vi "ics_ids_save_2D.vi"(0 "pixels":i32, 1 "filename":string, 3 "folder":path=path "D:/User/Sergey/ids_ics_trainer", 5 "Dwell":dbl, 7 "data":i32[][](array[numeric]), 9 "Range":dbl, 11 "error in":errorcluster) -> (4 "saved":bool, 15 "error out":errorcluster)   [LabVIEW 2009]
panel:
  out "text":string
  in  "scale I":i32=1
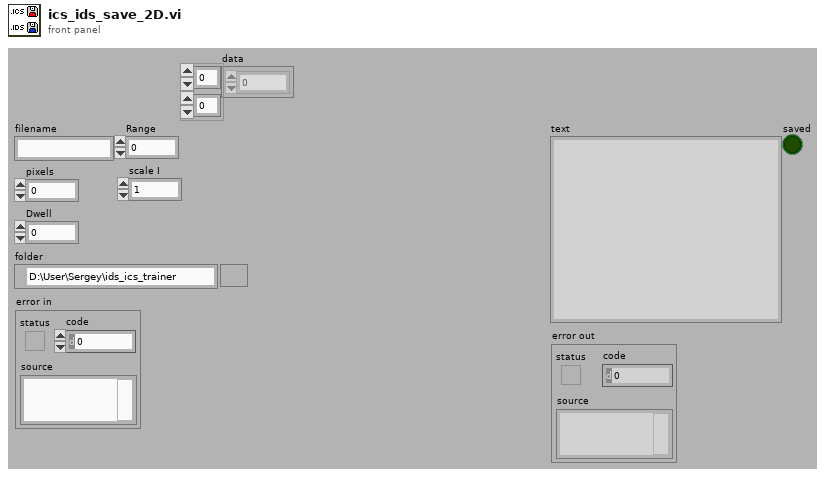
[diagram p1: front panel]
types:
  T1 = enum16{"open", "replace", "create", "open or create", "replace or create", "replace or create with confirmation"}
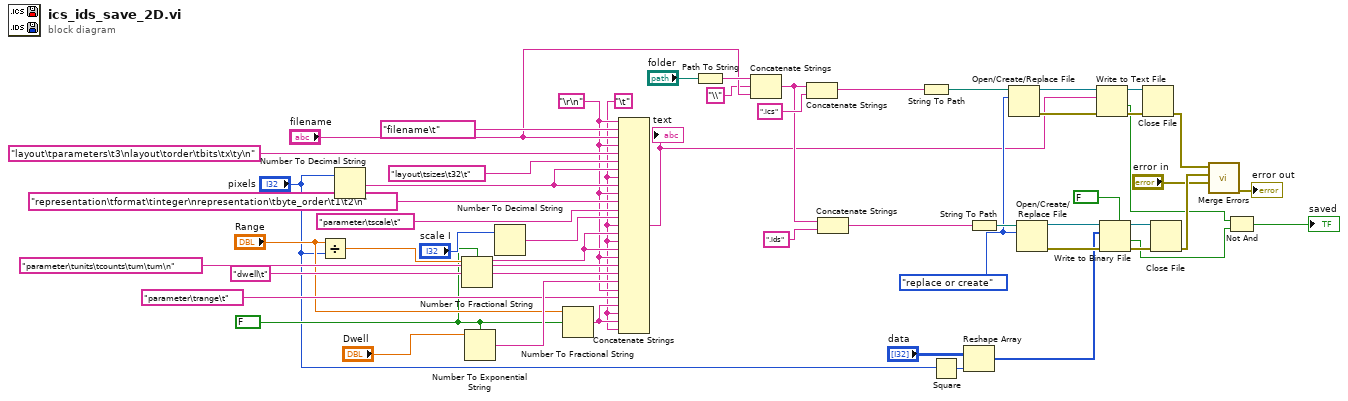
[diagram p0: block diagram]
diagram:
  w10 = FALSE ("use system decimal point (T)")
  w29 = T1."replace or create" ("operation (0:open)")
  w11 = "\t"
  w31 = "\r\n"
  n1 = Divide(x="Range", y="pixels") -> (x/y=w46:dbl)
  n2 = Number To Decimal String(number="pixels") -> (decimal integer string=w51:string)  [unwired: 1 in]
  n3 = Number To Fractional String(use system decimal point (T)=w10, number=w46) -> (F-format string=w45:string)  [unwired: 2 in]
  n4 = Number To Exponential String(number="Dwell", 1:w10) -> (E-format string=w40:string)  [unwired: 2 in]
  n5 = Number To Decimal String(number="scale I") -> (decimal integer string=w47:string)  [unwired: 1 in]
  n6 = Number To Fractional String(use system decimal point (T)=w10, number="Range") -> (F-format string=w12:string)  [unwired: 2 in]
  n7 = Concatenate Strings(w31, "filename\t" ("string"), "filename", w31, "layout\tparameters\t3\nlayout\torder\tbits\tx\ty\n" ("string"), "layout\tsizes\t32\t" ("string"), w51, w11, w51, w31, "representation\tformat\tinteger\nrepresentation\tbyte_order\t1\t2\n" ("string"), "parameter\tscale\t" ("string"), w47, w11, w45, w11, w45, w31, "parameter\tunits\tcounts\tum\tum\n" ("string"), "dwell\t" ("string"), w40, w31, "parameter\trange\t" ("string"), w12, w11, w12, w11) -> (w22:string)
  "text" <- w22
  n8 = Path To String(path="folder") -> (string=w35:string)
  n9 = Concatenate Strings(w35, "\\" ("string"), "filename") -> (w24:string)
  n10 = Concatenate Strings(w24, ".ics" ("string")) -> (w26:string)
  n11 = Concatenate Strings(w24, ".ids" ("string")) -> (w23:string)
  n12 = String To Path(string=w26) -> (path=w33:path)
  n13 = Square(x="pixels") -> (x^2=w16:i32)
  n14 = Reshape Array("data", w16) -> (w15:i32[])
  n15 = String To Path(string=w23) -> (path=w30:path)
  n16 = Open/Create/Replace File(file path (use dialog)=w33, operation (0:open)=w29) -> (refnum out=w37:refnum<file>, error out=w36:errorcluster)  [unwired: 4 in, 1 out]
  n17 = Open/Create/Replace File(file path (use dialog)=w30, operation (0:open)=w29) -> (refnum out=w19:refnum<file>, error out=w18:errorcluster)  [unwired: 4 in, 1 out]
  n18 = Write to Text File(file (use dialog)=w37, text=w22, error in=w36) -> (refnum out=w39:refnum<file>, cancelled=w5:bool, error out=w38:errorcluster)  [unwired: 1 in]
  n19 = Write to Binary File(file (use dialog)=w19, data=w15, error in=w18, 5:FALSE ("prepend array or string size? (T)")) -> (refnum out=w20:refnum<file>, cancelled=w4:bool, error out=w21:errorcluster)  [unwired: 2 in]
  n20 = Close File(refnum=w39, error in=w38) -> (error out=w9:errorcluster)  [unwired: 1 out]
  n21 = Close File(refnum=w20, error in=w21) -> (error out=w8:errorcluster)  [unwired: 1 out]
  n22 = call <vilib>:"Merge Errors.vi"("error in 3 (no error)"="error in", "error in 2 (no error)"=w8, "error in 1 (no error)"=w9) -> ("error out"=→"error out":errorcluster)  [unwired: 4 in]
  n23 = Not And(1:w4, 2:w5) -> (0:→"saved":bool)
